vi "Controller Write UINT16.vi"(8 "error in (no error)":errorcluster, 10 "Values":u16[](array[numeric]), 11 "Variables":refnum<k21>[](array[refnum])) -> (0 "error out":errorcluster)   [LabVIEW 2011, in "Controller VIs.lvlib"]
doc: "Writes a vector of unsigned integer 8-bit (byte) I/O variables."
uses:
  Controller VIs.lvlib
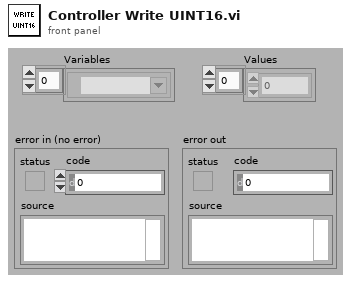
[diagram p1: front panel]
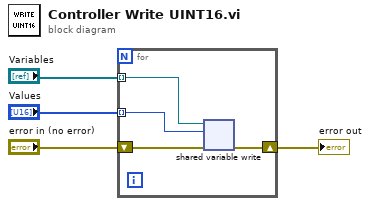
[diagram p0: block diagram]
diagram:
  n1 = for {
    tunnel: "Values" -> [w8] mode=indexing
    tunnel: "Variables" -> [w7] mode=indexing
    shift-right: [w5] -> w3
    shift-left: "error in (no error)" -> [w6]
    n2 = shared-variable-write(w7, w6, w8) -> (w5:errorcluster)  [unwired: 1 out]
  }
  "error out" <- w3
